vi "collectCI1_img.vi"() -> (0 "Avg cts/s":dbl, 1 "recorded samples":i32, 2 "wrap":i32)   [LabVIEW 2013]
uses:
  <vilib>/DAQmx/read.llb/DAQmx Read (Counter 1D U32 1Chan NSamp).vi
  <vilib>/DAQmx/miscellaneous.llb/DAQmx Fill In Error Info.vi
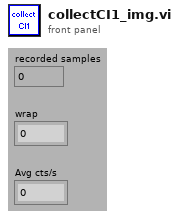
[diagram p1: front panel]
types:
  T1 = typedef "LVRectTypeDef.ctl" = cluster{"Left":i16, "Top":i16, "Right":i16, "Bottom":i16}
  T2 = cluster{"Xpixels":i32, "Vxminref":dbl, "Vxmaxref":dbl, "P":dbl, "Ypixels":i32, "Vyminref":dbl, "Vymaxref":dbl, "srate":sgl, "sAOxy":i32, "timeout":dbl, "type":string, "date":string, "time":string, "Colormap":u16, "Drawing Mode":u16, "Scanning Mode":u16, "square pixels":bool, "square matrix":bool, "Xpixels Img":i32, "Vx-min Img":dbl, "VX-max Img":dbl, "Ypixels Img":i32, "Vy-min Img":dbl, "Vy-max Img ":dbl, "Angle Img":dbl, "autoshutter":bool, "finite":bool, "cont":bool, "wavdet":bool, "measpoints":i32, "avpp":i32, "bufferAO":i32, "bufferAI":i32, "CH1":bool, "CH2":bool, "X":bool, "Y":bool, "Ip":bool, "Vp":bool, "starttick":u32, "waveform":path, "Vx-ref":dbl, "Vy-ref":dbl, "refreshrate":dbl, "refreshbuffer":i32, "tt_cycles":i32, "motorref":refnum<k7>, "mirrorswitch":refnum<k7>, "sample mode":i32, "maxbufferAI":i32, "sampletreshold":dbl, "srateAODO":sgl, "bin":sgl, "Pel":sgl, "Angle draw":dbl, "srate Img":sgl, "ROIimg_plotbounds":T1, "auto OD":bool, "ODfilt":u16, "reset AO_DO":bool}
  T3 = cluster{" CI1":refnum<k21>, "E_CI1":errorcluster}
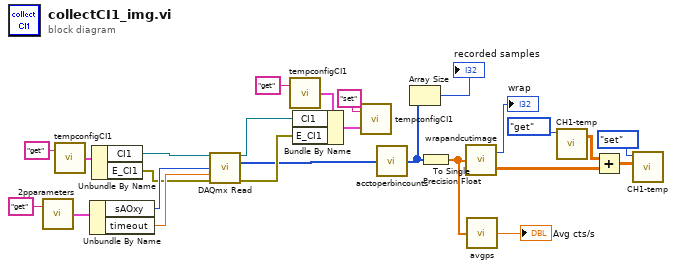
[diagram p0: block diagram]
diagram:
  n1 = call "2pparameters.vi"("command"="get") -> ("Params out"=w23:T2)  [unwired: 1 in]
  n2 = call "tempconfigCI1.vi"("command"="get") -> ("Temp Config out"=w17:T3)  [unwired: 1 in]
  n3 = Unbundle By Name(w23) -> ("sAOxy"=w24:i32, "timeout"=w25:dbl)
  n4 = Unbundle By Name(w17) -> ("CI1"=w18:refnum<k21>, "E_CI1"=w19:errorcluster)
  n5 = call-poly <vilib>:"DAQmx Read.vi"("task/channels in"=w18, "number of samples per channel"=w24, "timeout"=w25, "error in"=w19) -> ("task out"=w20:refnum<k21>, "data"=w1:u32[], "error out"=w21:errorcluster)  [unwired: 9 in]
  n6 = call "tempconfigCI1.vi"("command"="get") -> ("Temp Config out"=w15:T3)  [unwired: 1 in]
  n7 = Bundle By Name(cluster=w15, "CI1"=w20, "E_CI1"=w21) -> (w12:T3)
  n8 = call "tempconfigCI1.vi"("Temp Config in"=w12, "command"="set") -> ()  [unwired: 1 out]
  n9 = call "acctoperbincounts.vi"("accumulative counts"=w1) -> ("counts per bin"=w2:u32[])
  n10 = Array Size(array=w2) -> (size(s)=→"recorded samples":i32)
  n11 = To Single Precision Float(number=w2) -> (single precision float=w3:sgl[])
  n12 = call "wrapandcutimage.vi"("rasterscanned array"=w3) -> ("imagearray"=w6:sgl[][], "wrap"=→"wrap":i32)
  n13 = call "avgps.vi"("data"=w3) -> ("Avg cts/s"=→"Avg cts/s":dbl)
  n14 = call "CH1-temp.vi"("command"=enum16{"get", "set", "clear", "add row"}."get") -> ("array out"=w7:sgl[][])  [unwired: 3 in, 1 out]
  n15 = Add(x=w7, y=w6) -> (x+y=w8:sgl[][])
  n16 = call "CH1-temp.vi"("array in"=w8, "command"=enum16{"get", "set", "clear", "add row"}."set") -> ()  [unwired: 2 in, 2 out]
